vi "BuildRectangularScan_softturn.vi"(0 "VektorCluster":T2={"StartPunkt [m]"={"x"=-3.058577531863264e-05, "y"=1.835670165073038e-05}, "ZeilenIncrement [m]"={"x"=1.0229073667902263e-07, "y"=-4.894247696936301e-07}, "Zeile [m/s]"={"x"=0.21752211986383552, "y"=0.04546254963512117}, "Zeit/Zeile [s]"=0.000225}, 1 "ParameterCluster":T4={"x Pixel"=250, "Lines"=250, "Bidirektional"=TRUE, "AD-Frequency [Hz]"=4000000.0, "Galvo Cycle [s]"=1e-05, "Smartmovedelay [s]"=0.00119, "max.accel. [m/s^2]"=270000.0}) -> (2 "ScanSteuerung":T3(array[cluster])=[{"Zeitpunkt [s]"=0.0, "Wirkung"=enum."Abs", "Kanal"=enum."SMoveTime", "Wert (/s)"=0.0}, {"Zeitpunkt [s]"=0.0, "Wirkung"=enum."Abs", "Kanal"=enum."GalvoX", "Wert (/s)"=-3.058577531863264e-05}, {"Zeitpunkt [s]"=0.0, "Wirkung"=enum."Abs", "Kanal"=enum."GalvoY", "Wert (/s)"=1.835670165073038e-05}, {"Zeitpunkt [s]"=0.0, "Wirkung"=enum."Abs", "Kanal"=enum."Image1X", "Wert (/s)"=0.0}, {"Zeitpunkt [s]"=0.0, "Wirkung"=enum."Abs", "Kanal"=enum."Image1Y", "Wert (/s)"=0.0}, {"Zeitpunkt [s]"=0.0, "Wirkung"=enum."Abs", "Kanal"=enum."Digital", "Wert (/s)"=7.0}, {"Zeitpunkt [s]"=0.0, "Wirkung"=enum."LoopStart", "Kanal"=enum."Loop", "Wert (/s)"=49.0}, {"Zeitpunkt [s]"=0.0, "Wirkung"=enum."Inc", "Kanal"=enum."GalvoX", "Wert (/s)"=0.21752211986383552}, {"Zeitpunkt [s]"=0.0, "Wirkung"=enum."Inc", "Kanal"=enum."GalvoY", "Wert (/s)"=0.04546254963512117}, {"Zeitpunkt [s]"=0.0, "Wirkung"=enum."IncInc", "Kanal"=enum."GalvoX", "Wert (/s)"=0.0}, {"Zeitpunkt [s]"=0.0, "Wirkung"=enum."IncInc", "Kanal"=enum."GalvoY", "Wert (/s)"=0.0}, {"Zeitpunkt [s]"=0.0, "Wirkung"=enum."Inc", "Kanal"=enum."Image1X", "Wert (/s)"=444444.44444444444}, {"Zeitpunkt [s]"=0.00022275, "Wirkung"=enum."Inc", "Kanal"=enum."Image1X", "Wert (/s)"=0.0}, {"Zeitpunkt [s]"=0.000225, "Wirkung"=enum."Inc", "Kanal"=enum."Image1X", "Wert (/s)"=-2315789.47368421}, {"Zeitpunkt [s]"=0.000225, "Wirkung"=enum."Rel", "Kanal"=enum."Image1Y", "Wert (/s)"=1.0}, {"Zeitpunkt [s]"=0.00023, "Wirkung"=enum."Abs", "Kanal"=enum."Digital", "Wert (/s)"=5.0}, {"Zeitpunkt [s]"=0.00023, "Wirkung"=enum."IncInc", "Kanal"=enum."GalvoX", "Wert (/s)"=-146143.4081327828}, {"Zeitpunkt [s]"=0.00023, "Wirkung"=enum."IncInc", "Kanal"=enum."GalvoY", "Wert (/s)"=-32321.565855881716}, {"Zeitpunkt [s]"=0.00025, "Wirkung"=enum."IncInc", "Kanal"=enum."GalvoX", "Wert (/s)"=146143.4081327828}, {"Zeitpunkt [s]"=0.00025, "Wirkung"=enum."IncInc", "Kanal"=enum."GalvoY", "Wert (/s)"=32321.565855881716}, {"Zeitpunkt [s]"=0.00026775000000000003, "Wirkung"=enum."Inc", "Kanal"=enum."Image1X", "Wert (/s)"=0.0}, {"Zeitpunkt [s]"=0.00027, "Wirkung"=enum."Abs", "Kanal"=enum."Digital", "Wert (/s)"=7.0}, {"Zeitpunkt [s]"=0.00027, "Wirkung"=enum."LoopEnd", "Kanal"=enum."Loop", "Wert (/s)"=0.0}, {"Zeitpunkt [s]"=0.01323, "Wirkung"=enum."Inc", "Kanal"=enum."GalvoX", "Wert (/s)"=0.21752211986383552}, {"Zeitpunkt [s]"=0.01323, "Wirkung"=enum."Inc", "Kanal"=enum."GalvoY", "Wert (/s)"=0.04546254963512117}, {"Zeitpunkt [s]"=0.01323, "Wirkung"=enum."IncInc", "Kanal"=enum."GalvoX", "Wert (/s)"=0.0}, {"Zeitpunkt [s]"=0.01323, "Wirkung"=enum."IncInc", "Kanal"=enum."GalvoY", "Wert (/s)"=0.0}, {"Zeitpunkt [s]"=0.01323, "Wirkung"=enum."Inc", "Kanal"=enum."Image1X", "Wert (/s)"=444444.44444444444}, {"Zeitpunkt [s]"=0.013452750000000001, "Wirkung"=enum."Inc", "Kanal"=enum."Image1X", "Wert (/s)"=0.0}, {"Zeitpunkt [s]"=0.013455, "Wirkung"=enum."Inc", "Kanal"=enum."GalvoX", "Wert (/s)"=0.0}, {"Zeitpunkt [s]"=0.013455, "Wirkung"=enum."Inc", "Kanal"=enum."GalvoY", "Wert (/s)"=0.0}, {"Zeitpunkt [s]"=0.013455, "Wirkung"=enum."Abs", "Kanal"=enum."Digital", "Wert (/s)"=0.0}], 3 "Total time":dbl=0.013455, 4 "Line+Turn [s]":dbl=0.00027 format="%^#_6g")   [LabVIEW 2011]
panel:
  out "Galvo tun cycles":dbl=4.0
  out "turn [s] estimate":dbl=0.0004326610977478994
  out "Galvo too far":cluster{"x":dbl, "y":dbl}={"x"=1.087610599319179e-06, "y"=2.2731274817560613e-07}
  out "Galvo too late time":dbl=5.000000000000006e-06
  out "min Line+turn":dbl=0.000246633054887395
  out "exactTurn [s]":dbl=4.500000000000001e-05 format="%_6g"
  out "AD/pixel":u32=9
  out "Pixeltime":dbl=2.25e-06
  out "TotalPixel":u32=120
  out "validTotalCycles":u32=27
  out "ini":T1={"Bitsize-Zwischenbild"=5.5926e-07, "CCDmin"=7850.0, "CCDscale"=-10.85, "GalvoCycle"=1.2e-05, "Ext.AD-clock"=4000000.0, "Steps per optical density"=53.33} {"CCDscale" format="%.2f"; "CCDmin" format="%.2f"; "Bitsize-Zwischenbild" format="%.2e"}
  out "Zeit [s]/zeile":dbl=0.000225 min=0.0005 step=0.001 format="%^#_6g"
  out "min Galvocycles":u16=25
  # "Used Units: Pixels or meters in the intermediate image\nchanged May 18 2011\nTurn is extended until Pixel-clock is synchronous with GalvoClock\nuses the IncInc (aceleration) feature"
  # "looses 1 cycle as IncInc is changed at lineend and effect is 2 points later! (Inc is 1 later (next))\nneeds some clean up!"
  # "TriggerPin0: During Turn: High (Line End)\nTriggerPin1: During Frame: High (Frame Start)"
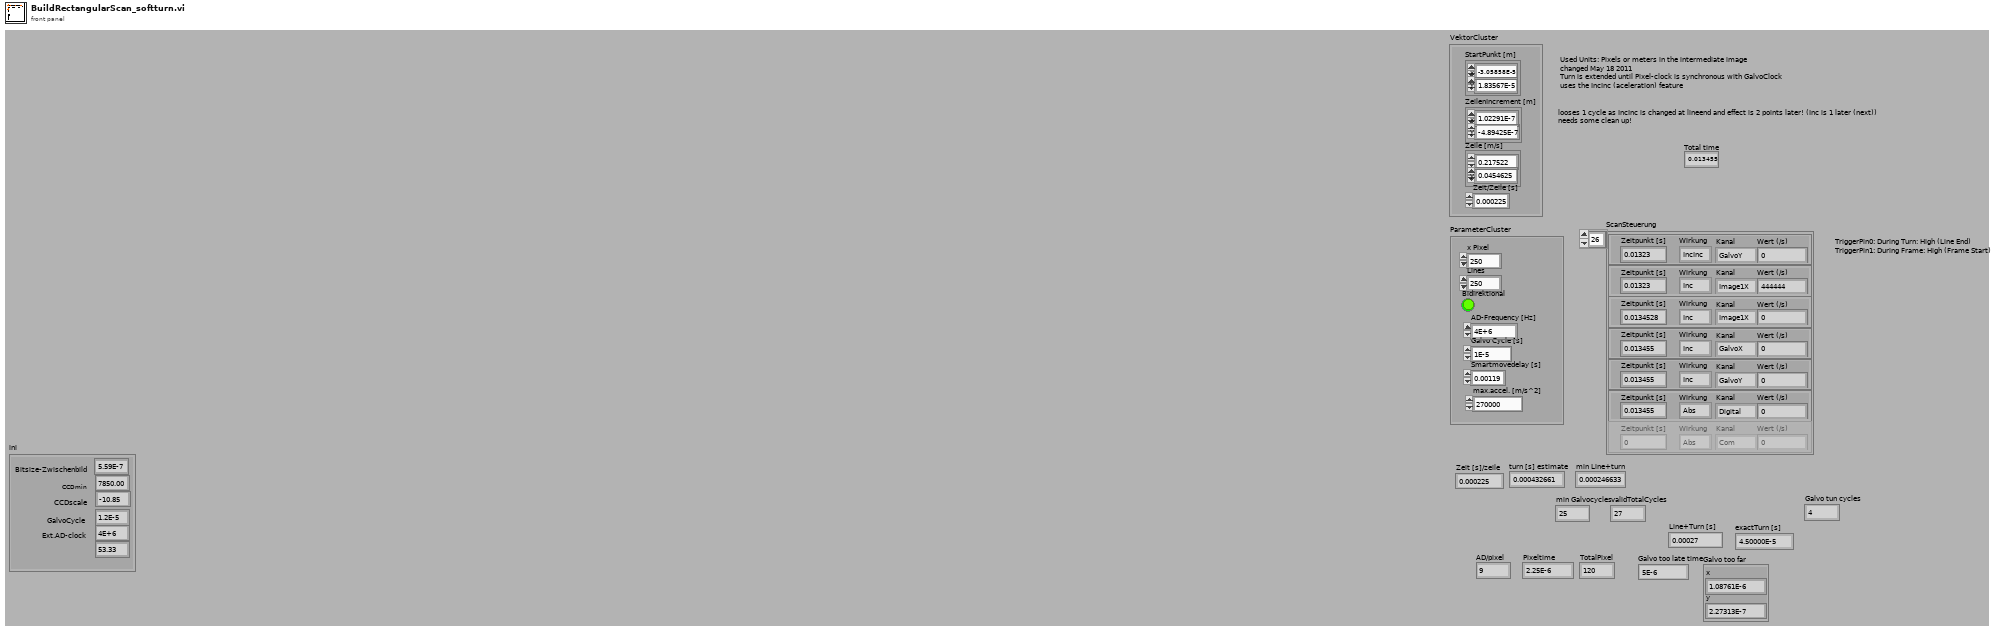
[diagram p1: front panel]
types:
  T1 = cluster{"Bitsize-Zwischenbild":dbl, "CCDmin":dbl, "CCDscale":dbl, "GalvoCycle":dbl, "Ext.AD-clock":dbl, "Steps per optical density":dbl}
  T2 = cluster{"StartPunkt [m]":cluster{"x":dbl, "y":dbl}, "ZeilenIncrement [m]":cluster{"x":dbl, "y":dbl}, "Zeile [m/s]":cluster{"x":dbl, "y":dbl}, "Zeit/Zeile [s]":dbl}
  T3 = cluster{"Zeitpunkt [s]":dbl, "Wirkung":enum16{"Abs", "Rel", "Inc", "IncInc", "LoopStart", "LoopEnd"}, "Kanal":enum16{"Com", "AnalogConfig", "AnalogValue", "GalvoX", "GalvoY", "Galvo3", "Galvo4", "Digital", "Free", "Loop", "SMoveTime", "Image1X", "Image1Y", "Image2X", "Image2Y"}, "Wert (/s)":dbl}[]
  T4 = cluster{"x Pixel":i32, "Lines":i32, "Bidirektional":bool, "AD-Frequency [Hz]":dbl, "Galvo Cycle [s]":dbl, "Smartmovedelay [s]":dbl, "max.accel. [m/s^2]":dbl}
  T5 = enum16{"Com", "AnalogConfig", "AnalogValue", "GalvoX", "GalvoY", "Galvo3", "Galvo4", "Digital", "Free", "Loop", "SMoveTime", "Image1X", "Image1Y", "Image2X", "Image2Y"}
  T6 = enum16{"Abs", "Rel", "Inc", "IncInc", "LoopStart", "LoopEnd"}
  T7 = typedef "ScanControl.ctl" = cluster{"Time [s]":dbl, "action":T8, "channel":T9, "value (/s)":dbl}[]
  T8 = typedef "ScanControl_Action.ctl" = enum16{"Abs", "Rel", "Inc", "IncInc", "LoopStart", "LoopEnd", "WaitTriggerRising"}
  T9 = typedef "ScanControl_Channel.ctl" = enum16{"Com", "AnalogConfig", "AnalogValue", "GalvoX", "GalvoY", "Galvo3", "Galvo4", "Digital", "Free", "Loop", "SMoveTime", "Image1X", "Image1Y", "Image2X", "Image2Y"}
  T10 = cluster{"Ende [s] AD+g raster":dbl, "Wirkung":enum16{"Abs", "Rel", "Inc", "IncInc", "LoopStart", "LoopEnd"}, "Kanal":enum16{"Com", "AnalogConfig", "AnalogValue", "GalvoX", "GalvoY", "Galvo3", "Galvo4", "Digital", "Free", "Loop", "SMoveTime", "Image1X", "Image1Y", "Image2X", "Image2Y"}, dbl}
  T11 = cluster{dbl, "Wirkung":enum16{"Abs", "Rel", "Inc", "IncInc", "LoopStart", "LoopEnd"}, "Kanal":enum16{"Com", "AnalogConfig", "AnalogValue", "GalvoX", "GalvoY", "Galvo3", "Galvo4", "Digital", "Free", "Loop", "SMoveTime", "Image1X", "Image1Y", "Image2X", "Image2Y"}, u8}
  T12 = cluster{dbl, "Wirkung":enum16{"Abs", "Rel", "Inc", "IncInc", "LoopStart", "LoopEnd"}, "Kanal":enum16{"Com", "AnalogConfig", "AnalogValue", "GalvoX", "GalvoY", "Galvo3", "Galvo4", "Digital", "Free", "Loop", "SMoveTime", "Image1X", "Image1Y", "Image2X", "Image2Y"}, dbl}
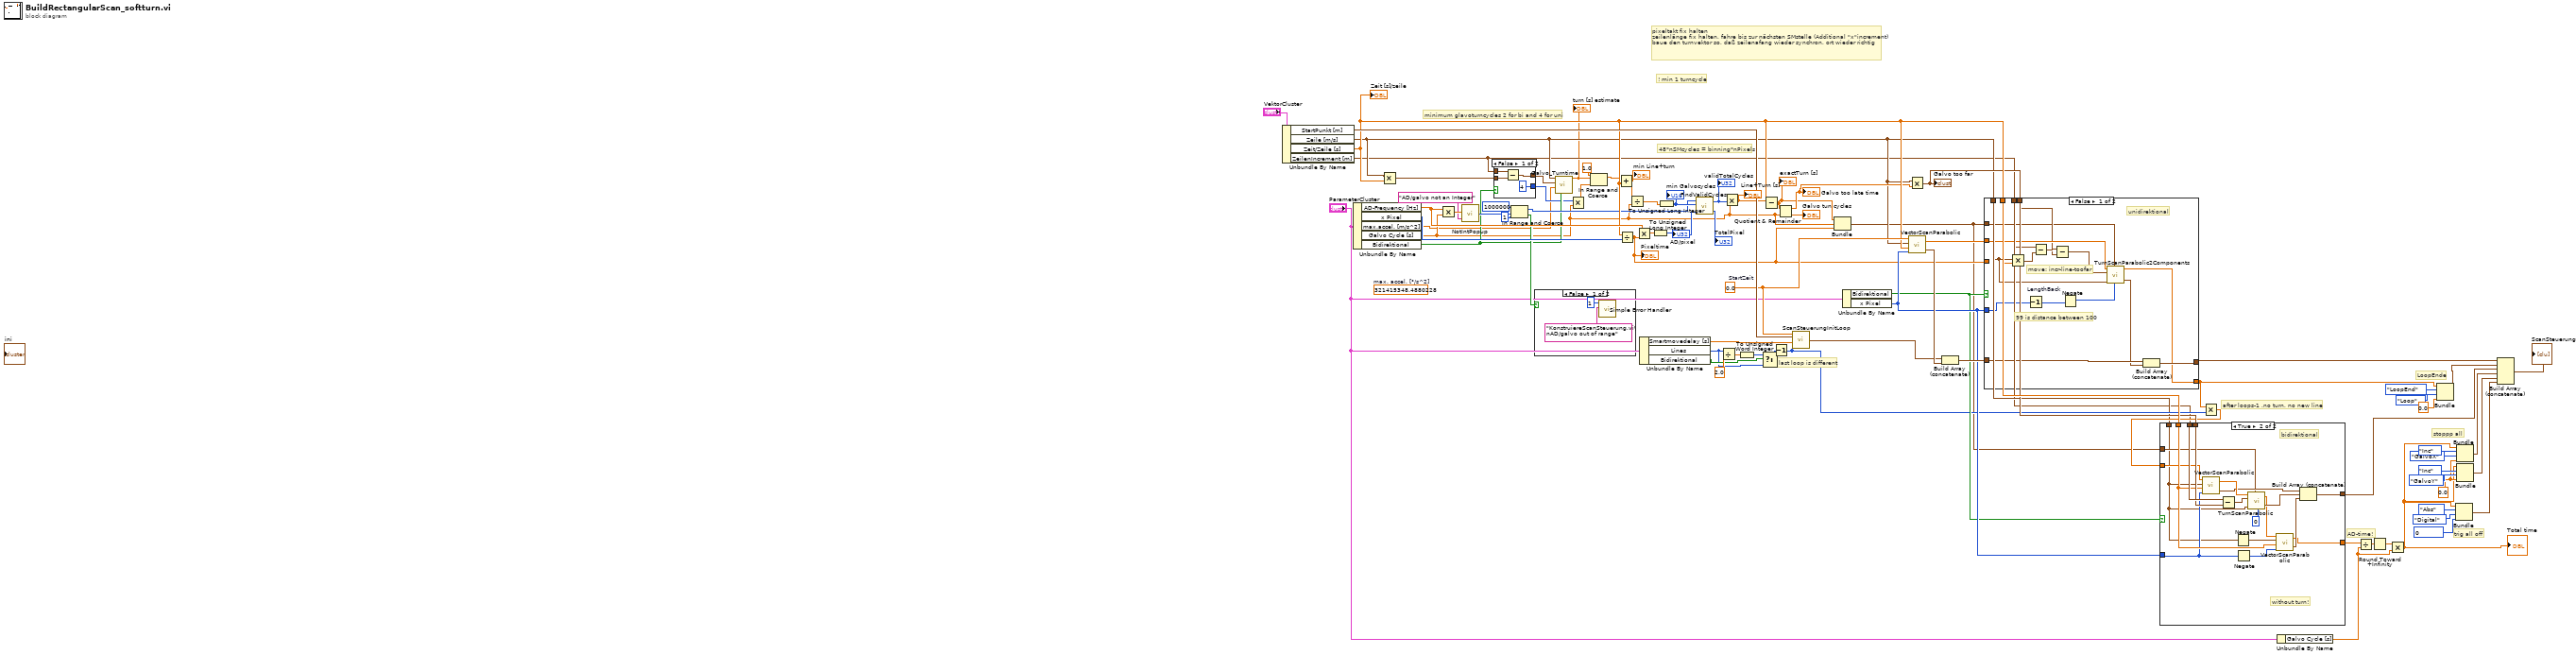
[diagram p0: block diagram]
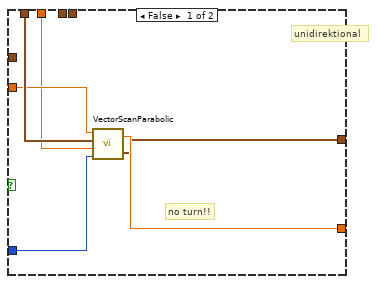
[diagram p3: hidden frame]
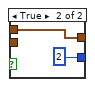
[diagram p4: hidden frame]
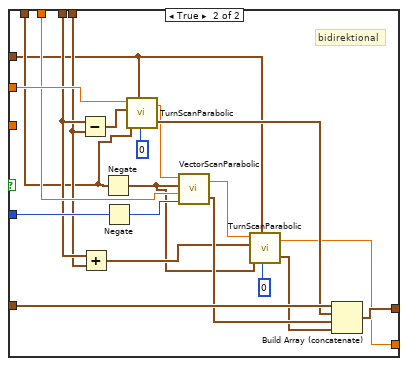
[diagram p5: hidden frame]
diagram:
  (unwired) 321415348.4880228  # max. accel. [°/s^2]
  w32 = 0.0
  w58 = 0.0  # StartZeit
  # "AD-time!"
  # "minimum glavoturncycles 2 for bi and 4 for uni"
  # "after loops-1 ,no turn, no new line"
  # "last loop is different"
  # "! min 1 turncycle"
  # "pixeltakt fix halten\nzeilenlänge fix halten, fahre bis zur nächsten SMstelle (Additional \"x\"increment)\nbaue den turnvektor so, daß zeilenafang wieder synchron, ort wieder richtig"
  # "48*nSMcycles = binning*nPixels"
  # "trig all off"
  # "stoppp all"
  # "LoopEnde"
  n1 = Unbundle By Name("VektorCluster") -> ("StartPunkt [m]"=w59:cluster{"x":dbl, "y":dbl}, "Zeile [m/s]"=w29:cluster{"x":dbl, "y":dbl}, "Zeit/Zeile [s]"=w52:dbl, "ZeilenIncrement [m]"=w28:cluster{"x":dbl, "y":dbl})
  "Zeit [s]/zeile" <- w52
  n2 = Unbundle By Name("ParameterCluster") -> ("AD-Frequency [Hz]"=w60:dbl, "x Pixel"=w67:i32, "max.accel. [m/s^2]"=w8:dbl, "Galvo Cycle [s]"=w18:dbl, "Bidirektional"=w30:bool)
  n3 = Multiply(x=w29, y=w52) -> (x*y=w26:cluster{"x":dbl, "y":dbl})
  n4 = Multiply(x=w60, y=w18) -> (x*y=w43:dbl)
  n5 = call "NotIntPopup.vi"("Err message"="AD/galvo not an Integer", "INT?"=w43) -> ("32bit integer"=w41:i32)  [unwired: 1 in]
  n6 = case shown="False" w30 {
    tunnel: w28 -> [w83 w85]
    tunnel: [w81 w85] -> w27
    tunnel: w26 -> [w82 _]
    tunnel: [4 2] -> w24
    frame False {
      n7 = Subtract(x=w83, y=w82) -> (x-y=w81:cluster{"x":dbl, "y":dbl})
    }
    frame True {
    }
  }
  n8 = In Range and Coerce(upper limit=1000000, x=w41, lower limit=1) -> (coerced(x)=w40:i32, In Range?=w37:bool)
  n9 = case shown="False" w37 {
    frame False {
      n10 = call <vilib>:"Simple Error Handler.vi"("error code (no error:0)"=1, "error source (\" \")"="KonstruiereScanSteuerung.vi\nAD/galvo out of range" ("Err message")) -> ()  [unwired: 2 in, 6 out]
    }
    frame True {
    }
  }
  n11 = call "Galvo_Turntime.vi"("bidirectional"=w30, "Maximal acceleration [m/s^2]"=w8, "delta x [m]"=w27, "start-speed [m/s]"=w29) -> ("duration [s]"=w7:dbl)  [unwired: 1 in, 6 out]
  "turn [s] estimate" <- w7
  n12 = Multiply(x=w24, y=w18) -> (x*y=w22:dbl)
  n13 = In Range and Coerce(upper limit=1.0, x=w7, lower limit=w22) -> (coerced(x)=w23:dbl)  [unwired: 1 out]
  n14 = Add(x=w23, y=w52) -> (x+y=w55:dbl)
  "min Line+turn" <- w55
  n15 = Divide(x=w52, y=w67) -> (x/y=w17:dbl)
  "Pixeltime" <- w17
  n16 = Divide(x=w55, y=w18) -> (x/y=w20:dbl)
  n17 = Multiply(x=w60, y=w17) -> (x*y=w61:dbl)
  n18 = Unbundle By Name("ParameterCluster") -> ("Smartmovedelay [s]"=w57:dbl, "Lines"=w10:i32, "Bidirektional"=w11:bool)
  n19 = To Unsigned Long Integer(number=w61) -> (unsigned 32bit integer=w62:u32)
  "AD/pixel" <- w62
  n20 = To Unsigned Long Integer(number=w20) -> (unsigned 32bit integer=w64:u32)
  "min Galvocycles" <- w64
  n21 = call "FindValidCycles.vi"("C (Fix)"=w62, "B (+x)"=w64, "A (Fix)"=w40) -> ("D"=→"TotalPixel":u32, "B Out"=w54:u32)
  "validTotalCycles" <- w54
  n22 = Divide(x=w10, y=2.0) -> (x/y=w13:dbl)
  n23 = Multiply(x=w18, y=w54) -> (x*y=w53:dbl)
  "Line+Turn [s]" <- w53
  n24 = To Unsigned Word Integer(number=w13) -> (unsigned 16bit integer=w12:u16)
  n25 = Select(t=w12, s=w11, f=w10) -> (s? t:f=w9:i32)
  n26 = Subtract(x=w53, y=w52) -> (x-y=w19:dbl)
  "exactTurn [s]" <- w19
  n27 = Decrement(x=w9) -> (x-1=w44:i32)
  n28 = Quotient & Remainder(x=w19, y=w18) -> (x-y*floor(x/y)=w50:dbl, floor(x/y)=→"Galvo tun cycles":dbl)
  "Galvo too late time" <- w50
  n29 = call "ScanSteuerungInitLoop.vi"("Loops"=w44, "Smartmovedelay [s]"=w57, "StartPunkt [m]"=w59, "StartZeit"=w58) -> ("ScanSteuerung"=w56:T7)
  n30 = Bundle(w19, "Galvo Cycle [s]"=w18, w17) -> (w16:cluster{dbl, "Galvo Cycle [s]":dbl, dbl})  [unwired: 1 out]
  n31 = Unbundle By Name("ParameterCluster") -> ("Bidirektional"=w48:bool, "x Pixel"=w49:i32)
  n32 = call "VectorScanParabolic.vi"("Pixel"=w49, "Zeit/zeile [s]"=w52, "Zeile [m/s]"=w29, "StartZeit"=w58) -> ("ScanSteuerung"=w66:T3, "EndZeit"=w65:dbl)
  n33 = Multiply(x=w29, y=w50) -> (x*y=w51:cluster{"x":dbl, "y":dbl})
  "Galvo too far" <- w51
  n34 = Build Array (concatenate)(w56, w66) -> (w79:T7)
  n35 = case shown="False" w48 {
    tunnel: w79 -> [w103 w124]
    tunnel: [w102 w123] -> w78
    tunnel: w29 -> [w90 w106]
    tunnel: w49 -> [w93 w122]
    tunnel: w28 -> [w101 w108]
    tunnel: w52 -> [w96 w111]
    tunnel: [w100 w116] -> w71
    tunnel: w65 -> [w97 w115]
    tunnel: w51 -> [w94 w107]
    tunnel: w17 -> [_ _]
    tunnel: w16 -> [w88 w104]
    frame False {
      # "99 is distance between 100"
      # "unidirektional"
      # "move: incr-line-toofar"
      n36 = Multiply(x=w90, y=w96) -> (x*y=w95:cluster{"x":dbl, "y":dbl})
      n37 = Decrement "LengthBack"(x=w93) -> (x-1=w92:i32)
      n38 = Subtract(x=w101, y=w95) -> (x-y=w99:cluster{"x":dbl, "y":dbl})
      n39 = Subtract(x=w99, y=w94) -> (x-y=w91:cluster{"x":dbl, "y":dbl})
      n40 = Negate(x=w92) -> (-x=w89:i32)
      n41 = call "TurnScanParabolic2Components.vi"("Start [s] AD raster"=w97, "TurnParameters"=w88, "deltaPosition [m]"=w91, "xPixel"=w89, "speed [m/s]"=w90) -> ("Ende [s] AD+g raster"=w100:dbl, "ScanSteuerung"=w98:T3)  [unwired: 2 in]
      n42 = Build Array (concatenate)(w103, w98) -> (w102:T7)
    }
    frame True {
      # "bidirektional"
      n43 = Subtract(x=w108, y=w107) -> (x-y=w110:cluster{"x":dbl, "y":dbl})
      n44 = Add(x=w108, y=w107) -> (x+y=w109:cluster{"x":dbl, "y":dbl})
      n45 = Negate(x=w106) -> (-x=w105:cluster{"x":dbl, "y":dbl})
      n46 = Negate(x=w122) -> (-x=w112:i32)
      n47 = call "TurnScanParabolic.vi"("xPixel"=0 ("Galvo"), "TurnParameters"=w104, "Zeile [m/s]"=w106, "corrZeilenIncrement [m]"=w110, "Start [s] AD raster"=w115) -> ("ScanSteuerung"=w120:T3, "Ende [s] AD+g raster"=w119:dbl)  [unwired: 1 in]
      n48 = call "VectorScanParabolic.vi"("Pixel"=w112, "Zeit/zeile [s]"=w111, "Zeile [m/s]"=w105, "StartZeit"=w119) -> ("ScanSteuerung"=w121:T3, "EndZeit"=w118:dbl)
      n49 = call "TurnScanParabolic.vi"("xPixel"=0 ("Galvo"), "TurnParameters"=w104, "Zeile [m/s]"=w105, "corrZeilenIncrement [m]"=w109, "Start [s] AD raster"=w118) -> ("ScanSteuerung"=w117:T3, "Ende [s] AD+g raster"=w116:dbl)  [unwired: 1 in]
      n50 = Build Array (concatenate)(w124, w120, w121, w117) -> (w123:T7)
    }
  }
  n51 = Multiply(x=w71, y=w44) -> (x*y=w47:dbl)
  n52 = case shown="True" w48 {
    tunnel: [w127 w148] -> w45
    tunnel: w29 -> [w130 w131]
    tunnel: w49 -> [w126 w134]
    tunnel: w28 -> [_ w140]
    tunnel: w52 -> [w125 w137]
    tunnel: [w128 w138] -> w5
    tunnel: w47 -> [w129 w136]
    tunnel: w51 -> [_ w139]
    tunnel: w16 -> [_ w132]
    frame False {
      # "no turn!!"
      # "unidirektional"
      n53 = call "VectorScanParabolic.vi"("Pixel"=w126, "Zeit/zeile [s]"=w125, "Zeile [m/s]"=w130, "StartZeit"=w129) -> ("ScanSteuerung"=w127:T3, "EndZeit"=w128:dbl)
    }
    frame True {
      # "without turn!"
      # "bidirektional"
      n54 = call "VectorScanParabolic.vi"("Pixel"=w134, "Zeit/zeile [s]"=w137, "Zeile [m/s]"=w131, "StartZeit"=w136) -> ("ScanSteuerung"=w133:T3, "EndZeit"=w135:dbl)
      n55 = Subtract(x=w140, y=w139) -> (x-y=w141:cluster{"x":dbl, "y":dbl})
      n56 = Negate(x=w131) -> (-x=w143:cluster{"x":dbl, "y":dbl})
      n57 = Negate(x=w134) -> (-x=w142:i32)
      n58 = call "TurnScanParabolic.vi"("xPixel"=0 ("Galvo"), "TurnParameters"=w132, "Zeile [m/s]"=w131, "corrZeilenIncrement [m]"=w141, "Start [s] AD raster"=w135) -> ("ScanSteuerung"=w146:T3, "Ende [s] AD+g raster"=w145:dbl)  [unwired: 1 in]
      n59 = call "VectorScanParabolic.vi"("Pixel"=w142, "Zeit/zeile [s]"=w137, "Zeile [m/s]"=w143, "StartZeit"=w145) -> ("ScanSteuerung"=w147:T3, "EndZeit"=w138:dbl)
      n60 = Build Array (concatenate)(w133, w146, w147) -> (w148:T3)
    }
  }
  n61 = Unbundle By Name("ParameterCluster") -> ("Galvo Cycle [s]"=w1:dbl)
  n62 = Divide(x=w5, y=w1) -> (x/y=w4:dbl)
  n63 = Round Toward +Infinity(x=w4) -> (ceil(x): smallest int >= x=w3:dbl)
  n64 = Multiply(x=w3, y=w1) -> (x*y=w6:dbl)
  "Total time" <- w6
  n65 = Bundle("Ende [s] AD+g raster"=w71, "Wirkung"=T6."LoopEnd", "Kanal"=T5."Loop", 0.0) -> (w76:T10)  [unwired: 1 out]
  n66 = Bundle(w6, "Wirkung"=T6."Abs", "Kanal"=T5."Digital", u8 0) -> (w68:T11)  [unwired: 1 out]
  n67 = Bundle(w6, "Wirkung"=T6."Inc", "Kanal"=T5."GalvoX", w32) -> (w46:T12)  [unwired: 1 out]
  n68 = Bundle(w6, "Wirkung"=T6."Inc", "Kanal"=T5."GalvoY", w32) -> (w72:T12)  [unwired: 1 out]
  n69 = Build Array (concatenate)(w78, w76, w45, w46, w72, w68) -> (→"ScanSteuerung":T7)
